vi "Treat Command.vi"(8 "error in (no error)":errorcluster, 11 "Channel in":refnum<class "SPARC4_Channel.lvclass">) -> (0 "error out":errorcluster, 3 "Channel out":refnum<class "SPARC4_Channel.lvclass">)   [LabVIEW 2018, in "SPARC4_Channel.lvclass"]
doc: "Treat the commando received from the control interface."
uses:
  SPARC4_Channel.lvclass
  State Machine/State Machine.lvclass
  Sim_CCD/Sim_CCD.lvclass
  RxTx/RxTx.lvclass
  Sim_Ixon_Ultra/Sim_Ixon_Ultra.lvclass
  C:/Users/Denis/Desktop/S4ACS/S4ACS/Sim_CCD/Sim_CCD.lvclass
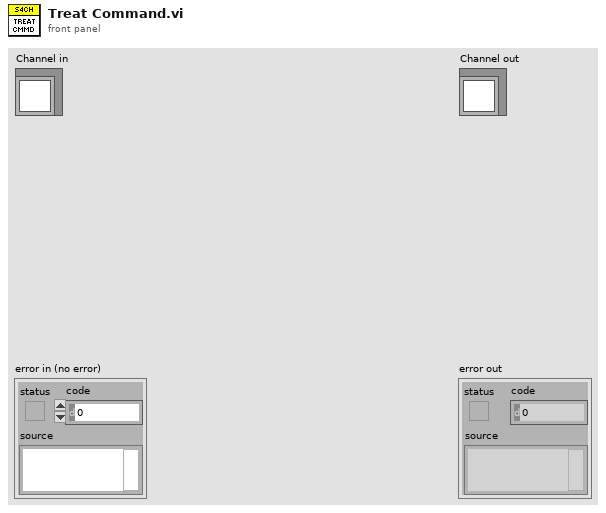
[diagram p1: front panel]
types:
  T1 = cluster{"FRAMES_DONE":u16, "CCD_STATUS":string, "CURRENT_TEMPERATURE":i16, "TEMPERATURE_STATUS":string, "FRAME_EXPOSURE_TIME":sgl, "SERIAL_NUMBER":u16, "ACQUIRING":bool, "POWER":bool}
  T2 = cluster{"CYCLES_DONE":u16, "LAST_IMAGE_NAME":string, "USED_DISK_SPACE":u16, "IMAGE_INDEX":u32, "SEQS_DONE":u16, "acquisition error":bool, "S4ICS comm attempts":u8}
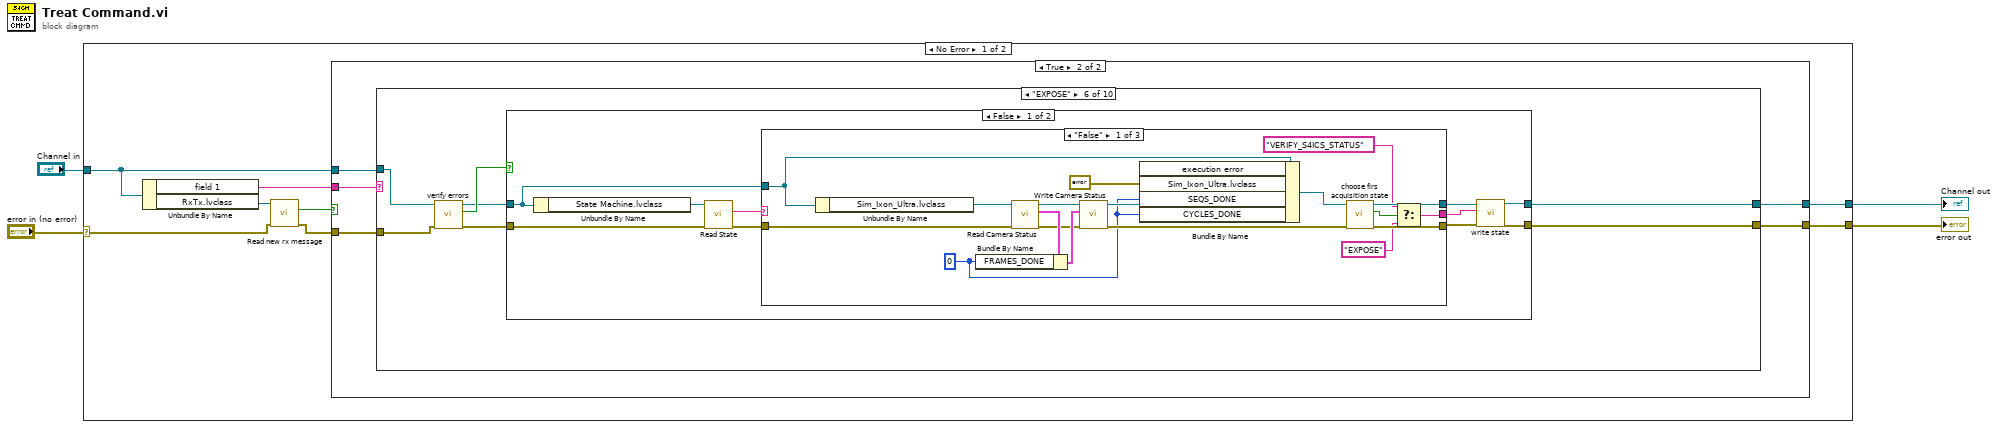
[diagram p0: block diagram]
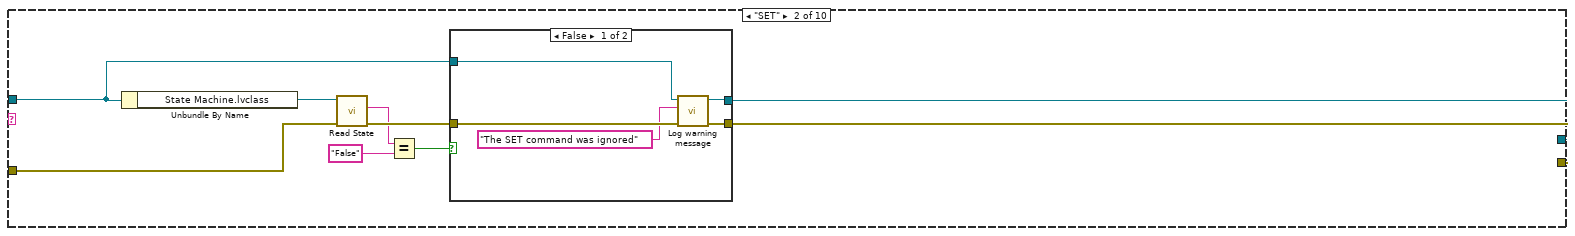
[diagram p4: hidden frame]
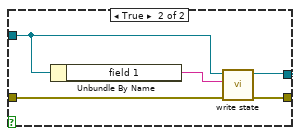
[diagram p5: hidden frame]
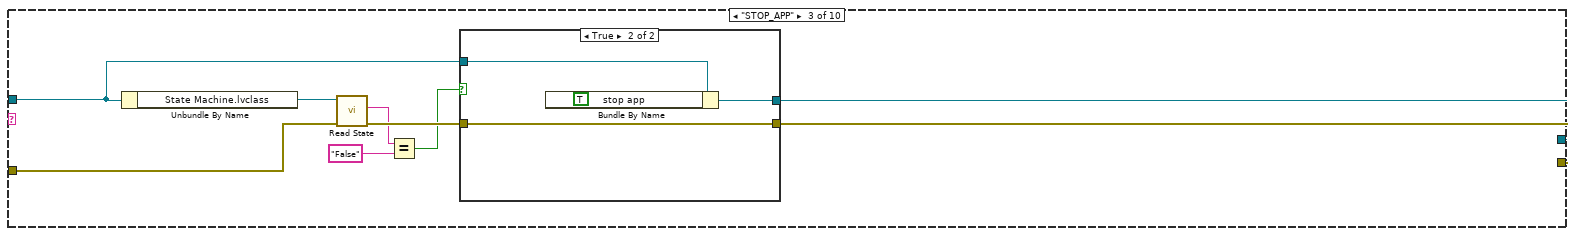
[diagram p6: hidden frame]
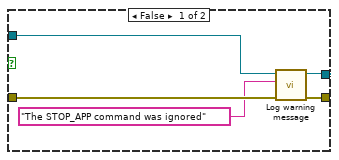
[diagram p7: hidden frame]
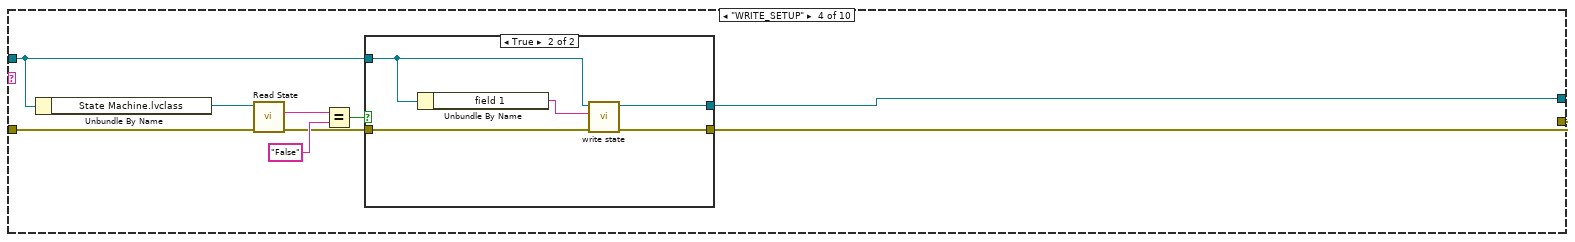
[diagram p8: hidden frame]
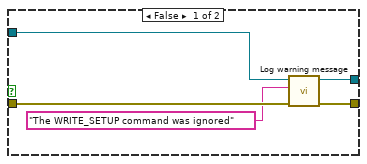
[diagram p9: hidden frame]
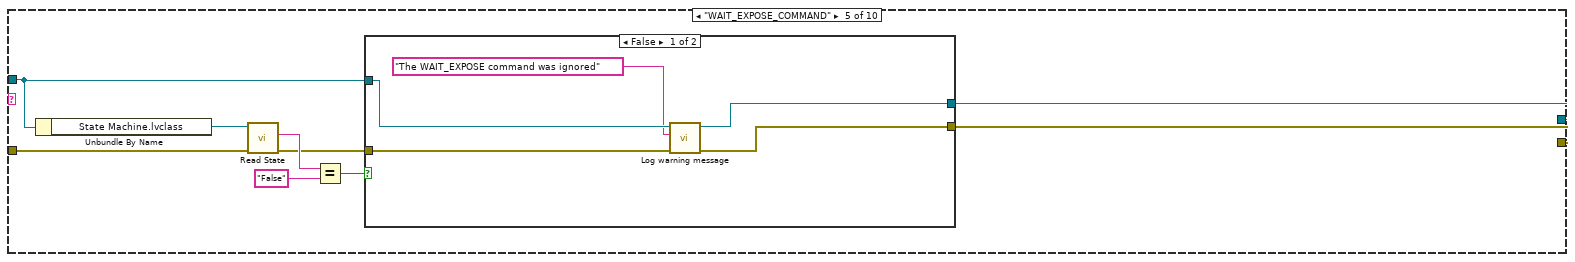
[diagram p10: hidden frame]
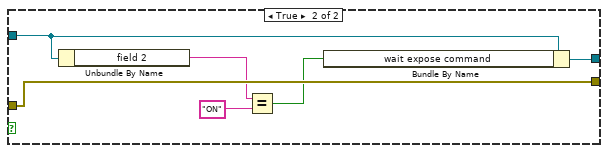
[diagram p11: hidden frame]
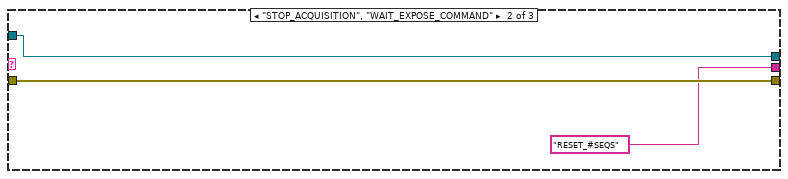
[diagram p12: hidden frame]
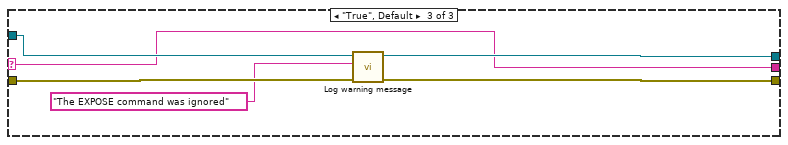
[diagram p13: hidden frame]
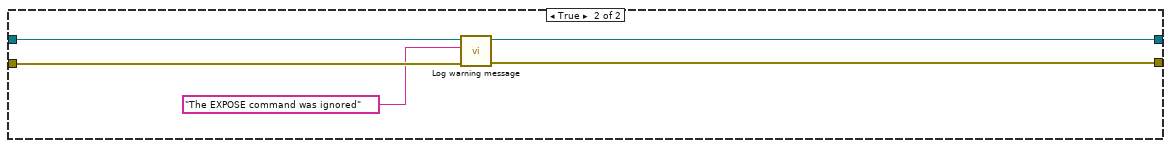
[diagram p14: hidden frame]
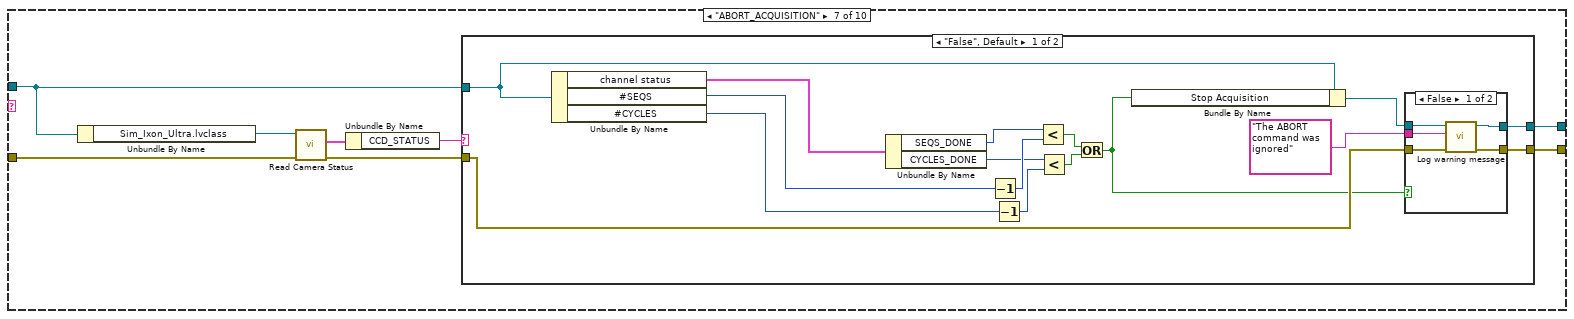
[diagram p15: hidden frame]
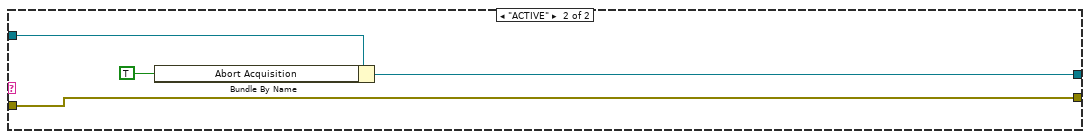
[diagram p17: hidden frame]
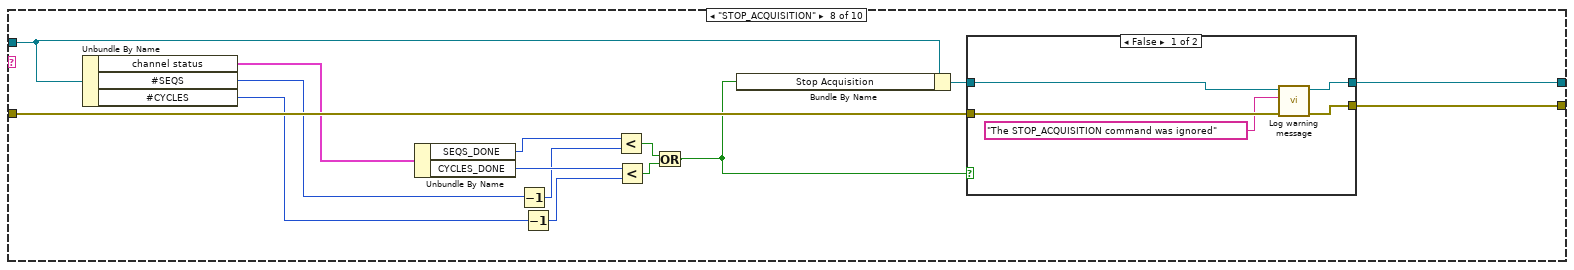
[diagram p18: hidden frame]
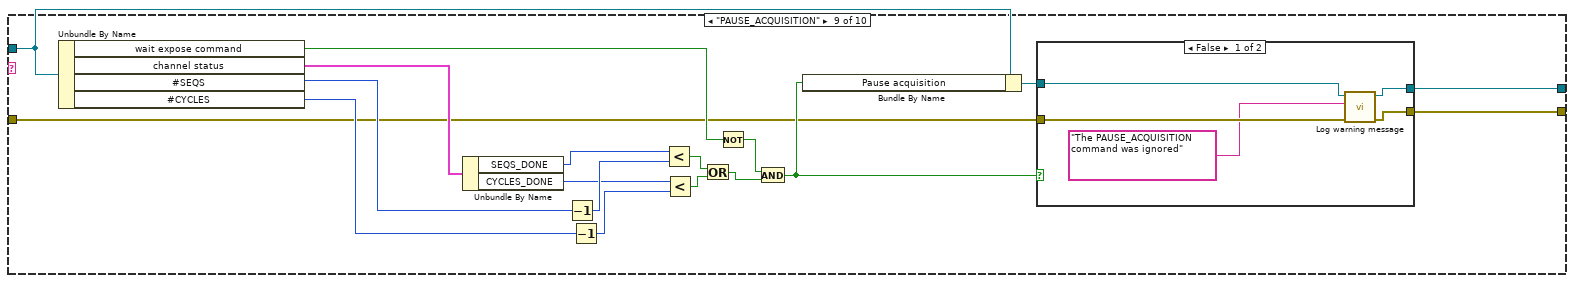
[diagram p20: hidden frame]
diagram:
  n1 = case shown="No Error" "error in (no error)" {
    selector: "error in (no error)" -> [w8 w247]
    tunnel: [w11 w247] -> w3
    tunnel: [w12 w246] -> w1
    tunnel: "Channel in" -> [w10 w246]
    frame No Error {
      n2 = Unbundle By Name(w10) -> ("field 1"=w5:string, "RxTx.lvclass"=w9:refnum<class "RxTx.lvclass">)
      n3 = call-dynamic "Read new rx message.vi"("error in (no error)"=w8, "RxTx in"=w9) -> ("error out"=w7:errorcluster, "new rx message"=w6:bool)  [unwired: 7 in, 1 out]
      n4 = case shown="True" w6 {
        tunnel: w7 -> [w13 w19]
        tunnel: [w14 w18] -> w12
        tunnel: [w13 w17] -> w11
        tunnel: w10 -> [w14 w16]
        tunnel: w5 -> [_ w15]
        frame False {
        }
        frame True {
          n5 = case shown="\"EXPOSE\"" w15 {
            tunnel: w16 -> [w21 w24 w43 w62 w81 w101 w154 w196 w221 w238]
            tunnel: [w21 w26 w45 w61 w79 w103 w153 w192 w220 w236] -> w18
            tunnel: w19 -> [w20 w27 w46 w65 w84 w102 w151 w194 w204 w237]
            tunnel: [w20 w25 w44 w60 w78 w104 w147 w191 w219 w235] -> w17
            frame "False", Default {
            }
            frame "SET" {
              n6 = Unbundle By Name(w24) -> ("State Machine.lvclass"=w29:refnum<class "State Machine.lvclass">)
              n7 = call-dynamic "Read State.vi"("error in (no error)"=w27, "State Machine in"=w29) -> ("error out"=w30:errorcluster, "State"=w23:string)  [unwired: 7 in, 1 out]
              n8 = Equal?(x=w23, y="False") -> (x = y?=w22:bool)
              n9 = case shown="False" w22 {
                tunnel: w30 -> [w35 w38]
                tunnel: [w33 w40] -> w26
                tunnel: [w34 w39] -> w25
                tunnel: w24 -> [w32 w37]
                frame False {
                  n10 = call "Log warning message.vi"("error in (no error)"=w35, "String"="The SET command was ignored", "Channel in"=w32) -> ("error out"=w34:errorcluster, "Channel out"=w33:refnum<class "SPARC4_Channel.lvclass">)  [unwired: 7 in]
                }
                frame True {
                  n11 = Unbundle By Name(w37) -> ("field 1"=w36:string)
                  n12 = call "write state.vi"("error in (no error)"=w38, "state"=w36, "Channel in"=w37) -> ("error out"=w39:errorcluster, "Channel out"=w40:refnum<class "SPARC4_Channel.lvclass">)  [unwired: 7 in]
                }
              }
            }
            frame "STOP_APP" {
              n13 = Unbundle By Name(w43) -> ("State Machine.lvclass"=w48:refnum<class "State Machine.lvclass">)
              n14 = call-dynamic "Read State.vi"("error in (no error)"=w46, "State Machine in"=w48) -> ("error out"=w49:errorcluster, "State"=w42:string)  [unwired: 7 in, 1 out]
              n15 = Equal?(x=w42, y="False") -> (x = y?=w41:bool)
              n16 = case shown="True" w41 {
                tunnel: w49 -> [w54 w58]
                tunnel: [w52 w56] -> w45
                tunnel: [w53 w58] -> w44
                tunnel: w43 -> [w51 w57]
                frame False {
                  n17 = call "Log warning message.vi"("error in (no error)"=w54, "String"="The STOP_APP command was ignored", "Channel in"=w51) -> ("error out"=w53:errorcluster, "Channel out"=w52:refnum<class "SPARC4_Channel.lvclass">)  [unwired: 7 in]
                }
                frame True {
                  n18 = Bundle By Name(cluster=w57, "stop app"=TRUE) -> (w56:refnum<class "SPARC4_Channel.lvclass">)
                }
              }
            }
            frame "WRITE_SETUP" {
              n19 = Unbundle By Name(w62) -> ("State Machine.lvclass"=w67:refnum<class "State Machine.lvclass">)
              n20 = call-dynamic "Read State.vi"("error in (no error)"=w65, "State Machine in"=w67) -> ("error out"=w63:errorcluster, "State"=w59:string)  [unwired: 7 in, 1 out]
              n21 = Equal?(x=w59, y="False") -> (x = y?=w64:bool)
              n22 = case shown="True" w64 {
                tunnel: w63 -> [w71 w77]
                tunnel: [w69 w75] -> w61
                tunnel: [w70 w76] -> w60
                tunnel: w62 -> [w72 w74]
                frame False {
                  n23 = call "Log warning message.vi"("error in (no error)"=w71, "String"="The WRITE_SETUP command was ignored", "Channel in"=w72) -> ("error out"=w70:errorcluster, "Channel out"=w69:refnum<class "SPARC4_Channel.lvclass">)  [unwired: 7 in]
                }
                frame True {
                  n24 = Unbundle By Name(w74) -> ("field 1"=w73:string)
                  n25 = call "write state.vi"("error in (no error)"=w77, "state"=w73, "Channel in"=w74) -> ("error out"=w76:errorcluster, "Channel out"=w75:refnum<class "SPARC4_Channel.lvclass">)  [unwired: 7 in]
                }
              }
            }
            frame "WAIT_EXPOSE_COMMAND" {
              n26 = Unbundle By Name(w81) -> ("State Machine.lvclass"=w86:refnum<class "State Machine.lvclass">)
              n27 = call-dynamic "Read State.vi"("error in (no error)"=w84, "State Machine in"=w86) -> ("error out"=w80:errorcluster, "State"=w83:string)  [unwired: 7 in, 1 out]
              n28 = Equal?(x=w83, y="False") -> (x = y?=w82:bool)
              n29 = case shown="False" w82 {
                tunnel: w81 -> [w91 w96]
                tunnel: w80 -> [w88 w97]
                tunnel: [w90 w94] -> w79
                tunnel: [w89 w97] -> w78
                frame False {
                  n30 = call "Log warning message.vi"("error in (no error)"=w88, "String"="The WAIT_EXPOSE command was ignored", "Channel in"=w91) -> ("error out"=w89:errorcluster, "Channel out"=w90:refnum<class "SPARC4_Channel.lvclass">)  [unwired: 7 in]
                }
                frame True {
                  n31 = Unbundle By Name(w96) -> ("field 2"=w92:string)
                  n32 = Equal?(x=w92, y="ON") -> (x = y?=w93:bool)
                  n33 = Bundle By Name(cluster=w96, "wait expose command"=w93) -> (w94:refnum<class "SPARC4_Channel.lvclass">)
                }
              }
            }
            frame "EXPOSE" {
              n34 = call "verify errors.vi"("error in (no error)"=w102, "Channel in"=w101) -> ("error out"=w98:errorcluster, "error"=w100:bool, "Channel out"=w99:refnum<class "SPARC4_Channel.lvclass">)  [unwired: 7 in]
              n35 = case shown="False" w100 {
                tunnel: [w107 w143] -> w104
                tunnel: w98 -> [w113 w145]
                tunnel: w99 -> [w111 w146]
                tunnel: [w108 w144] -> w103
                frame False {
                  n36 = Unbundle By Name(w111) -> ("State Machine.lvclass"=w114:refnum<class "State Machine.lvclass">)
                  n37 = call-dynamic "Read State.vi"("error in (no error)"=w113, "State Machine in"=w114) -> ("error out"=w110:errorcluster, "State"=w112:string)  [unwired: 7 in, 1 out]
                  n38 = case shown="\"False\"" w112 {
                    selector: w112 -> [_ _ w136]
                    tunnel: w111 -> [w126 w134 w141]
                    tunnel: w110 -> [w127 w135 w138]
                    tunnel: [w123 w134 w140] -> w109
                    tunnel: [w122 w135 w139] -> w106
                    tunnel: [w118 "RESET_#SEQS" w136] -> w105
                    frame "False" {
                      w115 = u16 0 ("CUBES_DONE")
                      n39 = Unbundle By Name(w126) -> ("Sim_Ixon_Ultra.lvclass"=w128:refnum<class "Sim_Ixon_Ultra.lvclass">)
                      n40 = call "Read Camera Status.vi"("error in (no error)"=w127, "CCDCamera in"=w128) -> ("error out"=w129:errorcluster, "camera status"=w131:T1, "CCDCamera out"=w132:refnum<class "Sim_Ixon_Ultra.lvclass">)  [unwired: 7 in]
                      n41 = Bundle By Name(cluster=w131, "FRAMES_DONE"=w115) -> (w130:T1)
                      n42 = call "Write Camera Status.vi"("error in (no error)"=w129, "camera status"=w130, "CCDCamera in"=w132) -> ("error out"=w121:errorcluster, "CCDCamera out"=w125:refnum<class "Sim_Ixon_Ultra.lvclass">)  [unwired: 7 in]
                      n43 = Bundle By Name(cluster=w126, "execution error"=errorcluster {"status"=FALSE, "code"=0, "source"=""}, "Sim_Ixon_Ultra.lvclass"=w125, "SEQS_DONE"=w115, "CYCLES_DONE"=w115) -> (w124:refnum<class "SPARC4_Channel.lvclass">)
                      n44 = call "choose firs acquisition state.vi"("error in (no error)"=w121, "Channel in"=w124) -> ("error out"=w122:errorcluster, "verify S4ICS status"=w117:bool, "Channel out"=w123:refnum<class "SPARC4_Channel.lvclass">)  [unwired: 7 in]
                      n45 = Select(t="VERIFY_S4ICS_STATUS" ("x"), s=w117, f="EXPOSE" ("x")) -> (s? t:f=w118:string)
                    }
                    frame "STOP_ACQUISITION", "WAIT_EXPOSE_COMMAND" {
                    }
                    frame "True", Default {
                      n46 = call "Log warning message.vi"("error in (no error)"=w138, "String"="The EXPOSE command was ignored", "Channel in"=w141) -> ("error out"=w139:errorcluster, "Channel out"=w140:refnum<class "SPARC4_Channel.lvclass">)  [unwired: 7 in]
                    }
                  }
                  n47 = call "write state.vi"("error in (no error)"=w106, "state"=w105, "Channel in"=w109) -> ("error out"=w107:errorcluster, "Channel out"=w108:refnum<class "SPARC4_Channel.lvclass">)  [unwired: 7 in]
                }
                frame True {
                  n48 = call "Log warning message.vi"("error in (no error)"=w145, "String"="The EXPOSE command was ignored" ("Message to log"), "Channel in"=w146) -> ("error out"=w143:errorcluster, "Channel out"=w144:refnum<class "SPARC4_Channel.lvclass">)  [unwired: 7 in]
                }
              }
            }
            frame "ABORT_ACQUISITION" {
              n49 = Unbundle By Name(w154) -> ("Sim_Ixon_Ultra.lvclass"=w150:refnum<class "Sim_Ixon_Ultra.lvclass">)
              n50 = call "Read Camera Status.vi"("error in (no error)"=w151, "CCDCamera in"=w150) -> ("error out"=w148:errorcluster, "camera status"=w152:T1)  [unwired: 7 in, 1 out]
              n51 = Unbundle By Name(w152) -> ("CCD_STATUS"=w149:string)
              n52 = case shown="\"False\", Default" w149 {
                tunnel: w154 -> [w164 w181]
                tunnel: [w160 w180] -> w153
                tunnel: w148 -> [w163 w178]
                tunnel: [w159 w178] -> w147
                frame "False", Default {
                  n53 = Unbundle By Name(w164) -> ("channel status"=w155:T2, "#SEQS"=w157:u32, "#CYCLES"=w156:u32)
                  n54 = Unbundle By Name(w155) -> ("SEQS_DONE"=w167:u16, "CYCLES_DONE"=w165:u16)
                  n55 = Decrement(x=w157) -> (x-1=w168:u32)
                  n56 = Decrement(x=w156) -> (x-1=w166:u32)
                  n57 = Less?(x=w167, y=w168) -> (x < y?=w170:bool)
                  n58 = Less?(x=w165, y=w166) -> (x < y?=w169:bool)
                  n59 = Or(x=w170, y=w169) -> (x .or. y?=w158:bool)
                  n60 = Bundle By Name(cluster=w164, "Stop Acquisition"=w158) -> (w161:refnum<class "SPARC4_Channel.lvclass">)
                  n61 = case shown="False" w158 {
                    tunnel: "The ABORT command was ignored" ("Message to log") -> [w175 _]
                    tunnel: w161 -> [w174 w176]
                    tunnel: [w173 w176] -> w160
                    tunnel: [w172 w177] -> w159
                    tunnel: w163 -> [w171 w177]
                    frame False {
                      n62 = call "Log warning message.vi"("error in (no error)"=w171, "String"=w175, "Channel in"=w174) -> ("error out"=w172:errorcluster, "Channel out"=w173:refnum<class "SPARC4_Channel.lvclass">)  [unwired: 7 in]
                    }
                    frame True {
                    }
                  }
                }
                frame "ACTIVE" {
                  n63 = Bundle By Name(cluster=w181, "Abort Acquisition"=TRUE) -> (w180:refnum<class "SPARC4_Channel.lvclass">)
                }
              }
            }
            frame "STOP_ACQUISITION" {
              n64 = Unbundle By Name(w196) -> ("channel status"=w182:T2, "#SEQS"=w183:u32, "#CYCLES"=w184:u32)
              n65 = Unbundle By Name(w182) -> ("SEQS_DONE"=w189:u16, "CYCLES_DONE"=w195:u16)
              n66 = Decrement(x=w183) -> (x-1=w188:u32)
              n67 = Decrement(x=w184) -> (x-1=w190:u32)
              n68 = Less?(x=w189, y=w188) -> (x < y?=w186:bool)
              n69 = Less?(x=w195, y=w190) -> (x < y?=w187:bool)
              n70 = Or(x=w186, y=w187) -> (x .or. y?=w185:bool)
              n71 = Bundle By Name(cluster=w196, "Stop Acquisition"=w185) -> (w193:refnum<class "SPARC4_Channel.lvclass">)
              n72 = case shown="False" w185 {
                tunnel: w193 -> [w201 w203]
                tunnel: w194 -> [w200 w202]
                tunnel: [w198 w203] -> w192
                tunnel: [w199 w202] -> w191
                frame False {
                  n73 = call "Log warning message.vi"("error in (no error)"=w200, "String"="The STOP_ACQUISITION command was ignored", "Channel in"=w201) -> ("error out"=w199:errorcluster, "Channel out"=w198:refnum<class "SPARC4_Channel.lvclass">)  [unwired: 7 in]
                }
                frame True {
                }
              }
            }
            frame "PAUSE_ACQUISITION" {
              n74 = Unbundle By Name(w221) -> ("wait expose command"=w216:bool, "channel status"=w205:T2, "#SEQS"=w207:u32, "#CYCLES"=w206:u32)
              n75 = Unbundle By Name(w205) -> ("SEQS_DONE"=w211:u16, "CYCLES_DONE"=w209:u16)
              n76 = Decrement(x=w207) -> (x-1=w212:u32)
              n77 = Decrement(x=w206) -> (x-1=w210:u32)
              n78 = Less?(x=w211, y=w212) -> (x < y?=w214:bool)
              n79 = Less?(x=w209, y=w210) -> (x < y?=w213:bool)
              n80 = Or(x=w214, y=w213) -> (x .or. y?=w208:bool)
              n81 = Not(x=w216) -> (.not. x?=w217:bool)
              n82 = And(x=w217, y=w208) -> (x .and. y?=w215:bool)
              n83 = Bundle By Name(cluster=w221, "Pause acquisition"=w215) -> (w218:refnum<class "SPARC4_Channel.lvclass">)
              n84 = case shown="False" w215 {
                tunnel: w218 -> [w226 w228]
                tunnel: w204 -> [w225 w227]
                tunnel: [w223 w228] -> w220
                tunnel: [w224 w227] -> w219
                frame False {
                  n85 = call "Log warning message.vi"("error in (no error)"=w225, "String"="The PAUSE_ACQUISITION command was ignored", "Channel in"=w226) -> ("error out"=w224:errorcluster, "Channel out"=w223:refnum<class "SPARC4_Channel.lvclass">)  [unwired: 7 in]
                }
                frame True {
                }
              }
            }
            frame "RESUME_ACQUISITION" {
              n86 = Unbundle By Name(w238) -> ("Pause acquisition"=w231:bool, "wait expose command"=w232:bool)
              n87 = Bundle By Name(cluster=w238, "Pause acquisition"=FALSE ("Acquisition control.Pause acquisition")) -> (w234:refnum<class "SPARC4_Channel.lvclass">)
              n88 = Not(x=w231) -> (.not. x?=w230:bool)
              n89 = Or(x=w230, y=w232) -> (x .or. y?=w229:bool)
              n90 = case shown="True" w229 {
                tunnel: w234 -> [w240 w245]
                tunnel: w237 -> [w239 w244]
                tunnel: [w240 w242] -> w236
                tunnel: [w239 w243] -> w235
                frame False {
                }
                frame True {
                  n91 = call "Log warning message.vi"("error in (no error)"=w244, "String"="The RESUME_ACQUISITION command was ignored", "Channel in"=w245) -> ("error out"=w243:errorcluster, "Channel out"=w242:refnum<class "SPARC4_Channel.lvclass">)  [unwired: 7 in]
                }
              }
            }
          }
        }
      }
    }
    frame Error {
    }
  }
  "error out" <- w3
  "Channel out" <- w1
